vi "Get Bank.vi"(9 "Bank Type":T1, 11 "?":T2=enum."Connector 3/Bank 3") -> (3 "Bank out":refnum<class "Bank.lvclass">)   [LabVIEW 2019, in "LRUTS FPGA IP.lvlib"]
uses:
  Bank/Bank.lvclass
  Bank List.ctl
  Bank/Bank Type.ctl
  Bank/FPGA IO Resources.ctl
  LRUTS FPGA IP.lvlib
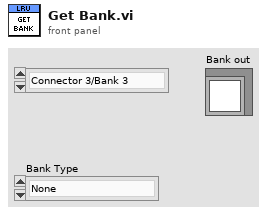
[diagram p1: front panel]
types:
  T1 = typedef "LRUTS FPGA IP.lvlib/Bank.lvclass/Bank Type.ctl" = enum16{"None", "Discrete Acquisition", "Discrete Generation", "PWM Acquisition", "PWM Generation"}
  T2 = typedef "LRUTS FPGA IP.lvlib/Bank List.ctl" = enum16{"Connector 0/Bank 0", "Connector 0/Bank 1", "Connector 0/Bank 2", "Connector 0/Bank 3", "Connector 1/Bank 0", "Connector 1/Bank 1", "Connector 1/Bank 2", "Connector 1/Bank 3", "Connector 2/Bank 0", "Connector 2/Bank 1", "Connector 2/Bank 2", "Connector 2/Bank 3", "Connector 3/Bank 0", "Connector 3/Bank 1", "Connector 3/Bank 2", "Connector 3/Bank 3"}
  T3 = typedef "LRUTS FPGA IP.lvlib/Bank.lvclass/FPGA IO Resources.ctl" = cluster{"DIO 0":refnum<k21>, "DIO 1":refnum<k21>, "DIO 2":refnum<k21>, "DIO 3":refnum<k21>, "DIO 4":refnum<k21>, "DIO 5":refnum<k21>, "DIO 6":refnum<k21>, "DIO 7":refnum<k21>}
  T4 = cluster{"DIO 0":refnum<k21>, "DIO 1":refnum<k21>, "DIO 2":refnum<k21>, "DIO 3":refnum<k21>, "DIO 4":refnum<k21>, "DIO 5":refnum<k21>, "DIO 6":refnum<k21>, "DIO 7":refnum<k21>}
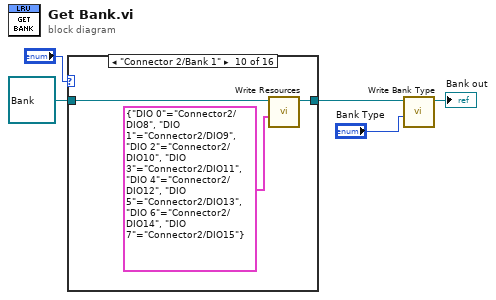
[diagram p0: block diagram]
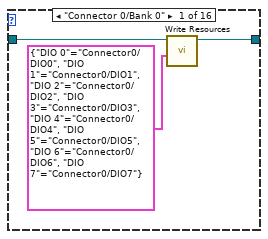
[diagram p2: hidden frame]
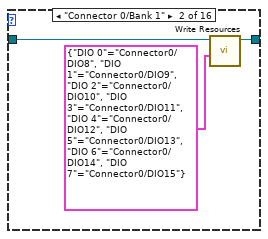
[diagram p3: hidden frame]
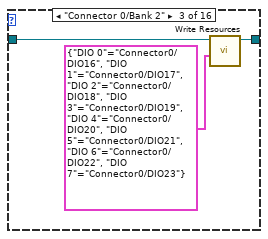
[diagram p4: hidden frame]
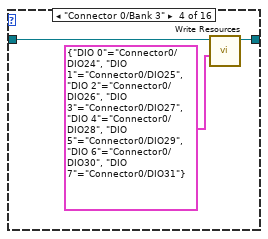
[diagram p5: hidden frame]
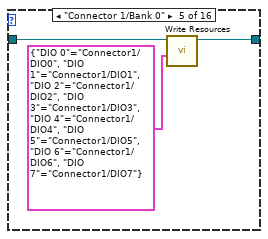
[diagram p6: hidden frame]
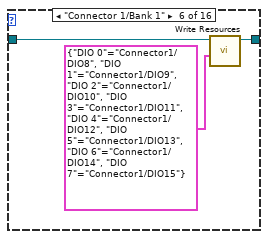
[diagram p7: hidden frame]
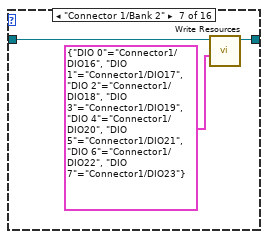
[diagram p8: hidden frame]
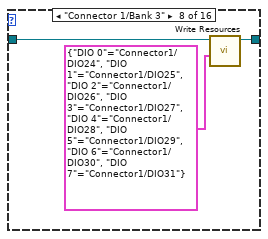
[diagram p9: hidden frame]
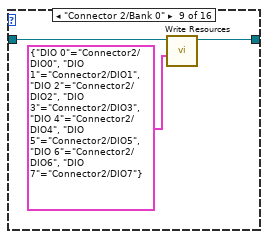
[diagram p10: hidden frame]
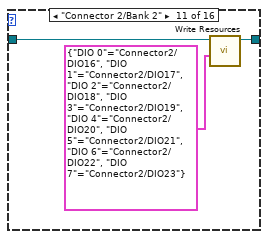
[diagram p11: hidden frame]
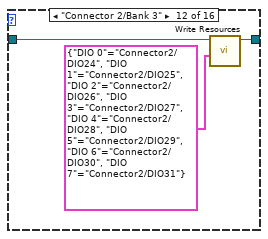
[diagram p12: hidden frame]
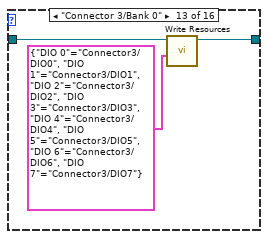
[diagram p13: hidden frame]
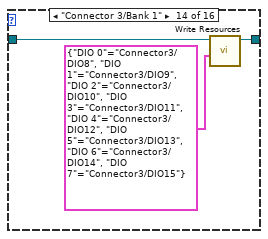
[diagram p14: hidden frame]
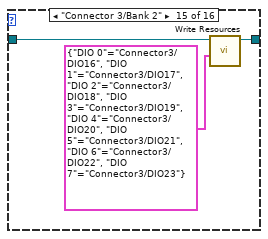
[diagram p15: hidden frame]
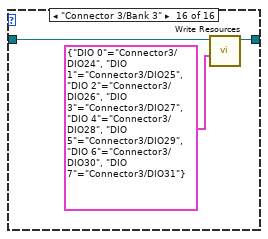
[diagram p16: hidden frame]
diagram:
  n1 = case shown="\"Connector 2/Bank 1\"" "?" {
    tunnel: refnum<class "Bank.lvclass"> refnum ("Bank in") -> [w8 w11 w14 w17 w20 w23 w26 w29 w32 w35 w38 w41 w44 w47 w50 w53]
    tunnel: [w7 w10 w13 w16 w19 w22 w25 w28 w31 w34 w37 w40 w43 w46 w49 w52] -> w3
    frame "Connector 0/Bank 0" {
      n2 = call "Write Resources.vi"("Resources"=T3 {"DIO 0"="Connector0/DIO0", "DIO 1"="Connector0/DIO1", "DIO 2"="Connector0/DIO2", "DIO 3"="Connector0/DIO3", "DIO 4"="Connector0/DIO4", "DIO 5"="Connector0/DIO5", "DIO 6"="Connector0/DIO6", "DIO 7"="Connector0/DIO7"}, "Bank in"=w8) -> ("Bank out"=w7:refnum<class "Bank.lvclass">)  [unwired: 9 in]
    }
    frame "Connector 0/Bank 1" {
      n3 = call "Write Resources.vi"("Resources"=T3 {"DIO 0"="Connector0/DIO8", "DIO 1"="Connector0/DIO9", "DIO 2"="Connector0/DIO10", "DIO 3"="Connector0/DIO11", "DIO 4"="Connector0/DIO12", "DIO 5"="Connector0/DIO13", "DIO 6"="Connector0/DIO14", "DIO 7"="Connector0/DIO15"}, "Bank in"=w11) -> ("Bank out"=w10:refnum<class "Bank.lvclass">)  [unwired: 9 in]
    }
    frame "Connector 0/Bank 2" {
      n4 = call "Write Resources.vi"("Resources"=T3 {"DIO 0"="Connector0/DIO16", "DIO 1"="Connector0/DIO17", "DIO 2"="Connector0/DIO18", "DIO 3"="Connector0/DIO19", "DIO 4"="Connector0/DIO20", "DIO 5"="Connector0/DIO21", "DIO 6"="Connector0/DIO22", "DIO 7"="Connector0/DIO23"}, "Bank in"=w14) -> ("Bank out"=w13:refnum<class "Bank.lvclass">)  [unwired: 9 in]
    }
    frame "Connector 0/Bank 3" {
      n5 = call "Write Resources.vi"("Resources"=T3 {"DIO 0"="Connector0/DIO24", "DIO 1"="Connector0/DIO25", "DIO 2"="Connector0/DIO26", "DIO 3"="Connector0/DIO27", "DIO 4"="Connector0/DIO28", "DIO 5"="Connector0/DIO29", "DIO 6"="Connector0/DIO30", "DIO 7"="Connector0/DIO31"}, "Bank in"=w17) -> ("Bank out"=w16:refnum<class "Bank.lvclass">)  [unwired: 9 in]
    }
    frame "Connector 1/Bank 0" {
      n6 = call "Write Resources.vi"("Resources"=T3 {"DIO 0"="Connector1/DIO0", "DIO 1"="Connector1/DIO1", "DIO 2"="Connector1/DIO2", "DIO 3"="Connector1/DIO3", "DIO 4"="Connector1/DIO4", "DIO 5"="Connector1/DIO5", "DIO 6"="Connector1/DIO6", "DIO 7"="Connector1/DIO7"}, "Bank in"=w20) -> ("Bank out"=w19:refnum<class "Bank.lvclass">)  [unwired: 9 in]
    }
    frame "Connector 1/Bank 1" {
      n7 = call "Write Resources.vi"("Resources"=T3 {"DIO 0"="Connector1/DIO8", "DIO 1"="Connector1/DIO9", "DIO 2"="Connector1/DIO10", "DIO 3"="Connector1/DIO11", "DIO 4"="Connector1/DIO12", "DIO 5"="Connector1/DIO13", "DIO 6"="Connector1/DIO14", "DIO 7"="Connector1/DIO15"}, "Bank in"=w23) -> ("Bank out"=w22:refnum<class "Bank.lvclass">)  [unwired: 9 in]
    }
    frame "Connector 1/Bank 2" {
      n8 = call "Write Resources.vi"("Resources"=T3 {"DIO 0"="Connector1/DIO16", "DIO 1"="Connector1/DIO17", "DIO 2"="Connector1/DIO18", "DIO 3"="Connector1/DIO19", "DIO 4"="Connector1/DIO20", "DIO 5"="Connector1/DIO21", "DIO 6"="Connector1/DIO22", "DIO 7"="Connector1/DIO23"}, "Bank in"=w26) -> ("Bank out"=w25:refnum<class "Bank.lvclass">)  [unwired: 9 in]
    }
    frame "Connector 1/Bank 3" {
      n9 = call "Write Resources.vi"("Resources"=T3 {"DIO 0"="Connector1/DIO24", "DIO 1"="Connector1/DIO25", "DIO 2"="Connector1/DIO26", "DIO 3"="Connector1/DIO27", "DIO 4"="Connector1/DIO28", "DIO 5"="Connector1/DIO29", "DIO 6"="Connector1/DIO30", "DIO 7"="Connector1/DIO31"}, "Bank in"=w29) -> ("Bank out"=w28:refnum<class "Bank.lvclass">)  [unwired: 9 in]
    }
    frame "Connector 2/Bank 0" {
      n10 = call "Write Resources.vi"("Resources"=T3 {"DIO 0"="Connector2/DIO0", "DIO 1"="Connector2/DIO1", "DIO 2"="Connector2/DIO2", "DIO 3"="Connector2/DIO3", "DIO 4"="Connector2/DIO4", "DIO 5"="Connector2/DIO5", "DIO 6"="Connector2/DIO6", "DIO 7"="Connector2/DIO7"}, "Bank in"=w32) -> ("Bank out"=w31:refnum<class "Bank.lvclass">)  [unwired: 9 in]
    }
    frame "Connector 2/Bank 1" {
      n11 = call "Write Resources.vi"("Resources"=T3 {"DIO 0"="Connector2/DIO8", "DIO 1"="Connector2/DIO9", "DIO 2"="Connector2/DIO10", "DIO 3"="Connector2/DIO11", "DIO 4"="Connector2/DIO12", "DIO 5"="Connector2/DIO13", "DIO 6"="Connector2/DIO14", "DIO 7"="Connector2/DIO15"}, "Bank in"=w35) -> ("Bank out"=w34:refnum<class "Bank.lvclass">)  [unwired: 9 in]
    }
    frame "Connector 2/Bank 2" {
      n12 = call "Write Resources.vi"("Resources"=T4 {"DIO 0"="Connector2/DIO16", "DIO 1"="Connector2/DIO17", "DIO 2"="Connector2/DIO18", "DIO 3"="Connector2/DIO19", "DIO 4"="Connector2/DIO20", "DIO 5"="Connector2/DIO21", "DIO 6"="Connector2/DIO22", "DIO 7"="Connector2/DIO23"}, "Bank in"=w38) -> ("Bank out"=w37:refnum<class "Bank.lvclass">)  [unwired: 9 in]
    }
    frame "Connector 2/Bank 3" {
      n13 = call "Write Resources.vi"("Resources"=T3 {"DIO 0"="Connector2/DIO24", "DIO 1"="Connector2/DIO25", "DIO 2"="Connector2/DIO26", "DIO 3"="Connector2/DIO27", "DIO 4"="Connector2/DIO28", "DIO 5"="Connector2/DIO29", "DIO 6"="Connector2/DIO30", "DIO 7"="Connector2/DIO31"}, "Bank in"=w41) -> ("Bank out"=w40:refnum<class "Bank.lvclass">)  [unwired: 9 in]
    }
    frame "Connector 3/Bank 0" {
      n14 = call "Write Resources.vi"("Resources"=T3 {"DIO 0"="Connector3/DIO0", "DIO 1"="Connector3/DIO1", "DIO 2"="Connector3/DIO2", "DIO 3"="Connector3/DIO3", "DIO 4"="Connector3/DIO4", "DIO 5"="Connector3/DIO5", "DIO 6"="Connector3/DIO6", "DIO 7"="Connector3/DIO7"}, "Bank in"=w44) -> ("Bank out"=w43:refnum<class "Bank.lvclass">)  [unwired: 9 in]
    }
    frame "Connector 3/Bank 1" {
      n15 = call "Write Resources.vi"("Resources"=T3 {"DIO 0"="Connector3/DIO8", "DIO 1"="Connector3/DIO9", "DIO 2"="Connector3/DIO10", "DIO 3"="Connector3/DIO11", "DIO 4"="Connector3/DIO12", "DIO 5"="Connector3/DIO13", "DIO 6"="Connector3/DIO14", "DIO 7"="Connector3/DIO15"}, "Bank in"=w47) -> ("Bank out"=w46:refnum<class "Bank.lvclass">)  [unwired: 9 in]
    }
    frame "Connector 3/Bank 2" {
      n16 = call "Write Resources.vi"("Resources"=T3 {"DIO 0"="Connector3/DIO16", "DIO 1"="Connector3/DIO17", "DIO 2"="Connector3/DIO18", "DIO 3"="Connector3/DIO19", "DIO 4"="Connector3/DIO20", "DIO 5"="Connector3/DIO21", "DIO 6"="Connector3/DIO22", "DIO 7"="Connector3/DIO23"}, "Bank in"=w50) -> ("Bank out"=w49:refnum<class "Bank.lvclass">)  [unwired: 9 in]
    }
    frame "Connector 3/Bank 3" {
      n17 = call "Write Resources.vi"("Resources"=T3 {"DIO 0"="Connector3/DIO24", "DIO 1"="Connector3/DIO25", "DIO 2"="Connector3/DIO26", "DIO 3"="Connector3/DIO27", "DIO 4"="Connector3/DIO28", "DIO 5"="Connector3/DIO29", "DIO 6"="Connector3/DIO30", "DIO 7"="Connector3/DIO31"}, "Bank in"=w53) -> ("Bank out"=w52:refnum<class "Bank.lvclass">)  [unwired: 9 in]
    }
  }
  n18 = call "Write Bank Type.vi"("Bank Type"="Bank Type", "Bank in"=w3) -> ("Bank out"=→"Bank out":refnum<class "Bank.lvclass">)  [unwired: 9 in]
